vi "BRig_RT__Case_Exp__sendData__endExp.vi"() -> ()   [LabVIEW 2014]
uses:
  <vilib>/WebDAVClient/Advanced/SessionHandle.ctl
  <vilib>/WebDAVClient/NI_WebDAV.lvlib
panel:
  in  "input_fileName_prefix":string
  in  "input_I_connected_webdav":bool
  in  "input_hComm_webdav":T1
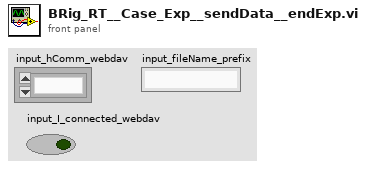
[diagram p1: front panel]
types:
  T1 = typedef "NI_WebDAV.lvlib/SessionHandle.ctl" = refnum<k1>
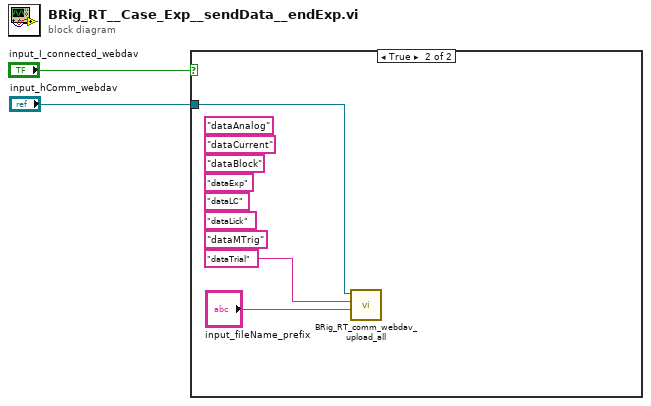
[diagram p0: block diagram]
diagram:
  n1 = case shown="True" "input_I_connected_webdav" {
    tunnel: "input_hComm_webdav" -> [_ w3]
    frame False {
    }
    frame True {
      (unwired) "dataAnalog" ("input_filename")
      (unwired) "dataMTrig" ("input_filename")
      (unwired) "dataLick" ("input_filename")
      (unwired) "dataLC" ("input_filename")
      (unwired) "dataExp" ("input_filename")
      (unwired) "dataBlock" ("input_filename")
      (unwired) "dataCurrent" ("input_filename")
      n2 = call "BRig_RT_comm_webdav_upload_all.vi"("input_fileName_prefix"="input_fileName_prefix", 10:"dataTrial" ("input_filename"), "input_hSession"=w3) -> ()  [unwired: 8 in, 1 out]
    }
  }
